vi "Ethernet Transmit.vi"(8 "error in (no error)":errorcluster, 9 "Timeout":i32=10000, 10 "Code":string="IP", 11 "TCP Connection Refnum in":refnum<k5>) -> (0 "error out":errorcluster, 3 "TCP Connection Refnum (dup)":refnum<k5>)   [LabVIEW 2019]
panel:
  # "VI Name: MB Serial Transmit.vi\nPurpose: Sends a Modbus message.\nReentrant because its caller is reentrant."
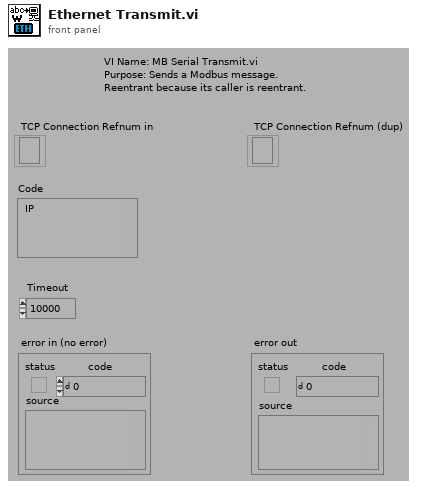
[diagram p1: front panel]
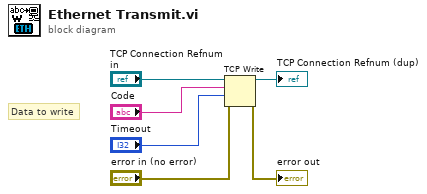
[diagram p0: block diagram]
diagram:
  # "Data to write"
  n1 = TCP Write(connection ID="TCP Connection Refnum in", data in="Code", error in (no error)="error in (no error)", 9:"Timeout") -> (connection ID out=→"TCP Connection Refnum (dup)":refnum<k5>, error out=→"error out":errorcluster)  [unwired: 1 out]
